vi "Initialize Transfer Groups.vi"(7 "component name":string, 8 "error in":errorcluster, 10 "Group Configurations":refnum<class "Group Configuration.lvclass">[](array[class]), 11 "RDMA Transceiver in":refnum<class "RDMA Transceiver.lvclass">) -> (0 "error out":errorcluster, 3 "RDMA Transceiver out":refnum<class "RDMA Transceiver.lvclass">)   [LabVIEW 2020, in "RDMA.lvlib" / "RDMA Transceiver.lvclass"]
doc: "Initializes all transfer groups"
uses:
  RDMA Transceiver.lvclass
  DSF Core.lvlibp/Classes/Configuration/Core/Group/Group Configuration.lvclass
  RDMA Transceiver.lvclass/RDMA Transceiver.ctl
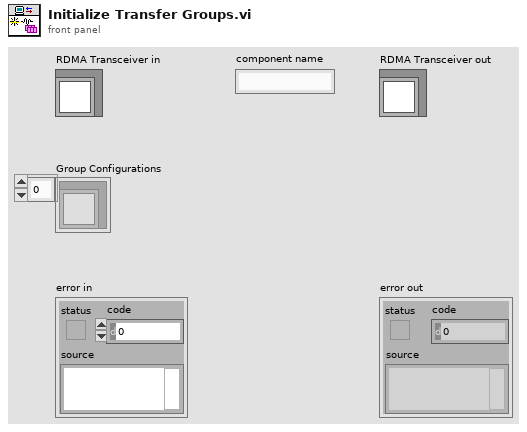
[diagram p1: front panel]
types:
  T1 = typedef "RDMA.lvlib/RDMA Transceiver.lvclass/Transfer Parameters.ctl" = cluster{"connected session":refnum<k21>, "listener session":refnum<k21>}
  T2 = cluster{"Transfer Configuration":refnum<class "Transfer Configuration.lvclass">, "group id":i32, "transfer id":i32, "transfer parameters":T1}[]
  T3 = typedef "RDMA.lvlib/RDMA Transceiver.lvclass/Transfer Group Parameters.ctl" = cluster{"transfers":T1[]}
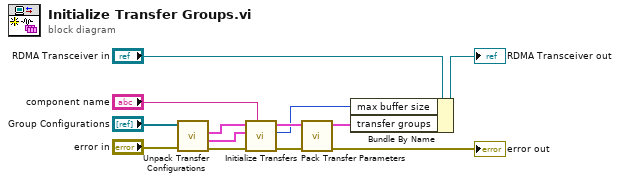
[diagram p0: block diagram]
diagram:
  n1 = call "Unpack Transfer Configurations.vi"("error in"="error in", "Group Configurations"="Group Configurations") -> ("error out"=w9:errorcluster, "Labeled RX Transfer Configurations"=w8:T2, "Labeled TX Transfer Configurations"=w11:T2)  [unwired: 7 in]
  n2 = call "Initialize Transfers.vi"("component name"="component name", "error in"=w9, "Labeled RX Transfer Configurations"=w8, "Labeled TX Transfer Configurations"=w11) -> ("error out"=w6:errorcluster, "max buffer size"=w2:i32, "Labeled Transfer Parameters"=w7:T2)  [unwired: 5 in]
  n3 = call "Pack Transfer Parameters.vi"("error in"=w6, "Labeled Transfer Parameters"=w7) -> ("dup error out"=→"error out":errorcluster, "Transfer Groups"=w1:T3[])  [unwired: 8 in]
  n4 = Bundle By Name(cluster="RDMA Transceiver in", "max buffer size"=w2, "transfer groups"=w1) -> (→"RDMA Transceiver out":refnum<class "RDMA Transceiver.lvclass">)
